vi "FindBlobs.vi"(10 "Vision Target":enum16{"Pegs", "Gears"}(ring), 11 "Image In":T2) -> (2 "Blob Data":T1, 3 "Image Out":T2)   [LabVIEW 2016]
uses:
  <vilib>/vision/Image Controls.llb/IMAQ Image.ctl
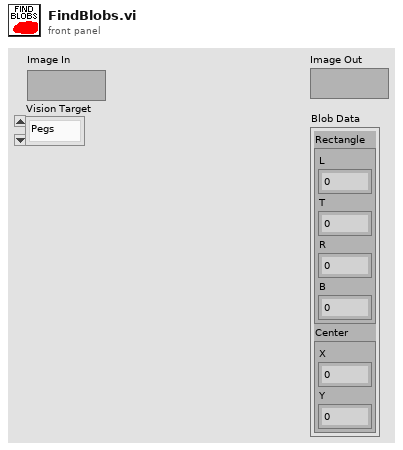
[diagram p1: front panel]
types:
  T1 = cluster{"Rectangle":cluster{"L":dbl, "T":dbl, "R":dbl, "B":dbl}, "Center":cluster{"X":dbl, "Y":dbl}}
  T2 = typedef "IMAQ Image.ctl" = refnum<image>
  T3 = typedef "Particle Parameters" = i32
  T4 = cluster{"Numeric":dbl, "Numeric":dbl, "Numeric":dbl, "Numeric":dbl}
  T5 = cluster{"Left":dbl, "Top":dbl, "Right":dbl, "Bottom":dbl}
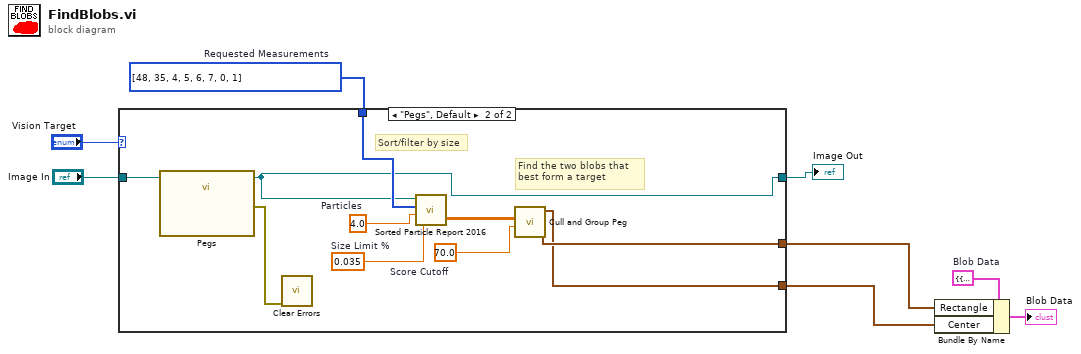
[diagram p0: block diagram]
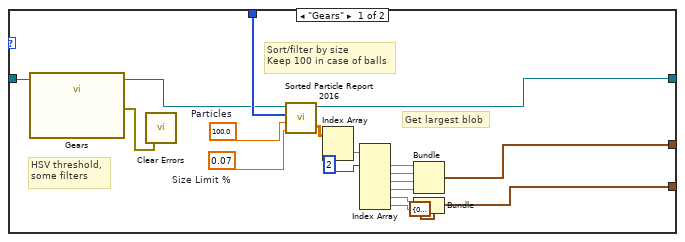
[diagram p2: hidden frame]
diagram:
  w4 = T1 {"Rectangle"={"L"=0.0, "T"=0.0, "R"=0.0, "B"=0.0}, "Center"={"X"=0.0, "Y"=0.0}}  # Blob Data
  w7 = T3[] [48, 35, 4, 5, 6, 7, 0, 1] items=["Center of Mass X", "Center of Mass Y", "First Pixel X", "First Pixel Y", "Bounding Rect Left", "Bounding Rect Top", "Bounding Rect Right", "Bounding Rect Bottom", "Max Feret Diameter Start X", "Max Feret Diameter Start Y", "Max Feret Diameter End X", "Max Feret Diameter End Y", "Max Horiz. Segment Length Left", "Max Horiz. Segment Length Right", "Max Horiz. Segment Length Row", "-", "Bounding Rect Width", "Bounding Rect Height", "Bounding Rect Diagonal", "Perimeter", "Convex Hull Perimeter", "Holes' Perimeter", "Max Feret Diameter", "Equivalent Ellipse Major Axis", "Equivalent Ellipse Minor Axis", "Equivalent Ellipse Minor Axis (Feret)", "Equivalent Rect Long Side", "Equivalent Rect Short Side", "Equivalent Rect Diagonal", "Equivalent Rect Short Side (Feret)", "Average Horiz. Segment Length", "Average Vert. Segment Length", "Hydraulic Radius", "Waddel Disk Diameter", "-", "Area", "Holes' Area", "Particle & Holes' Area", "Convex Hull Area", "Image Area", "-", "Number of Holes", "Number of Horiz. Segments", "Number of Vert. Segments", "-", "Orientation", "Max Feret Diameter Orientation", "-", "% Area/Image Area", "% Area/(Particle & Holes' Area)", "Ratio of Equivalent Ellipse Axes", "Ratio of Equivalent Rect Sides", "-", "Elongation Factor", "Compactness Factor", "Heywood Circularity Factor", "Type Factor", "-", "Sum X", "Sum Y", "Sum XX", "Sum XY", "Sum YY", "Sum XXX", "Sum XXY", "Sum XYY", "Sum YYY", "-", "Moment of Inertia XX", "Moment of Inertia XY", "Moment of Inertia YY", "Moment of Inertia XXX", "Moment of Inertia XXY", "Moment of Inertia XYY", "Moment of Inertia YYY", "Norm. Moment of Inertia XX", "Norm. Moment of Inertia XY", "Norm. Moment of Inertia YY", "Norm. Moment of Inertia XXX", "Norm. Moment of Inertia XXY", "Norm. Moment of Inertia XYY", "Norm. Moment of Inertia YYY", "Hu Moment 1", "Hu Moment 2", "Hu Moment 3", "Hu Moment 4", "Hu Moment 5", "Hu Moment 6", "Hu Moment 7"]  # Requested Measurements
  n1 = case shown="\"Pegs\", Default" "Vision Target" {
    tunnel: w7 -> [w22 w34]
    tunnel: [w9 w30] -> w1
    tunnel: "Image In" -> [w25 w28]
    tunnel: [w21 w27] -> w5
    tunnel: [w10 w31] -> w2
    frame "Gears" {
      w24 = 100.0  # Particles
      w23 = 0.07  # Size Limit %
      # "Get largest blob"
      # "Sort/filter by size\nKeep 100 in case of balls"
      # "HSV threshold,\nsome filters"
      n2 = call "Gears"("Image In"=w25) -> ("Image Out"=w21:T2, "error out"=w26:errorcluster)  [unwired: 25 in]
      n3 = call <vilib>:"Clear Errors.vi"("error in (no error)"=w26) -> ()  [unwired: 5 in, 2 out]
      n4 = call "Sorted Particle Report 2016.vi"("Min Area Size %"=w23, "Particle Count Limit"=w24, "Pixel Measurements"=w22, "Image in"=w21) -> ("Sorted Data"=w20:dbl[][])  [unwired: 1 out]
      n5 = Index Array(array=w20) -> (element=w19:dbl[])  [unwired: 2 in]
      n6 = Index Array(array=w19, index #1=2 ("index")) -> (element #1=w17:dbl, element #2=w16:dbl, element #3=w15:dbl, element #4=w14:dbl, element #5=w12:dbl, element #6=w13:dbl)  [unwired: 5 in]
      n7 = Bundle("Numeric"=w17, "Numeric"=w16, "Numeric"=w15, "Numeric"=w14) -> (w10:T4)  [unwired: 1 in]
      n8 = Bundle(cluster=cluster{"X":dbl, "Y":dbl} {"X"=0.0, "Y"=0.0} ("input cluster"), "X"=w12, "Y"=w13) -> (w9:cluster{"X":dbl, "Y":dbl})
    }
    frame "Pegs", Default {
      w32 = 70.0  # Score Cutoff
      w36 = 4.0  # Particles
      w35 = 0.035  # Size Limit %
      # "Find the two blobs that \nbest form a target"
      # "Sort/filter by size"
      n9 = call "Pegs"("Image In"=w28) -> ("Image Out"=w27:T2, "error out"=w29:errorcluster)  [unwired: 25 in]
      n10 = call <vilib>:"Clear Errors.vi"("error in (no error)"=w29) -> ()  [unwired: 5 in, 2 out]
      n11 = call "Sorted Particle Report 2016.vi"("Min Area Size %"=w35, "Particle Count Limit"=w36, "Pixel Measurements"=w34, "Image in"=w27) -> ("Sorted Data"=w33:dbl[][])  [unwired: 1 out]
      n12 = call "Cull and Group Peg.vi"("Score Cutoff"=w32, "Sorted Data"=w33) -> ("Rect"=w31:T5, "Center"=w30:cluster{"X":dbl, "Y":dbl})  [unwired: 6 in, 2 out]
    }
  }
  "Image Out" <- w5
  n13 = Bundle By Name(cluster=w4, "Rectangle"=w2, "Center"=w1) -> (→"Blob Data":T1)
